vi "UpdateStatistics.vi"(8 "error in (no error)":errorcluster, 10 "Statistics":cluster{"OK":i32, "NG":i32}, 11 "WebSocket in":refnum<class "WebSocket.lvclass">) -> (0 "error out":errorcluster, 3 "WebSocket out":refnum<class "WebSocket.lvclass">)   [LabVIEW 2019, in "WebSocket.lvlib" / "WebSocket.lvclass"]
uses:
  WebSocket.lvclass
  ec31b149-a411-4443-9d0d-94b6aa8f2f4f.vi
  <vilib>/JDP Science/JSONtext/Variant to JSON Text.vi
  <vilib>/JDP Science/JSONtext/LVClass Serializer/JSONtext LVClass Serializer.lvclass
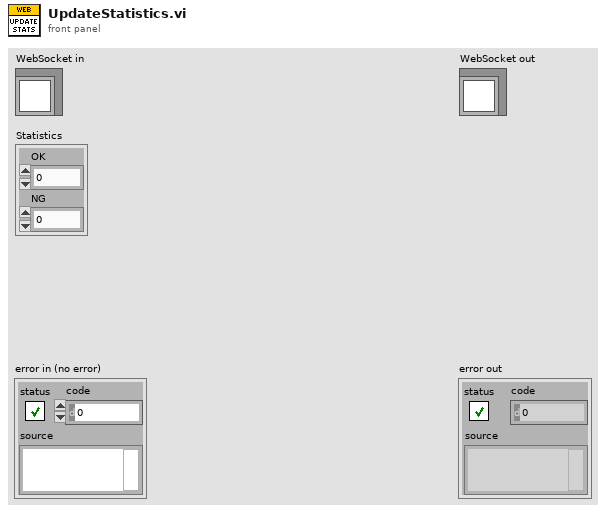
[diagram p1: front panel]
types:
  T1 = cluster{"type":string, "count":cluster{"ok":i32, "ng":i32, "yield":dbl}}
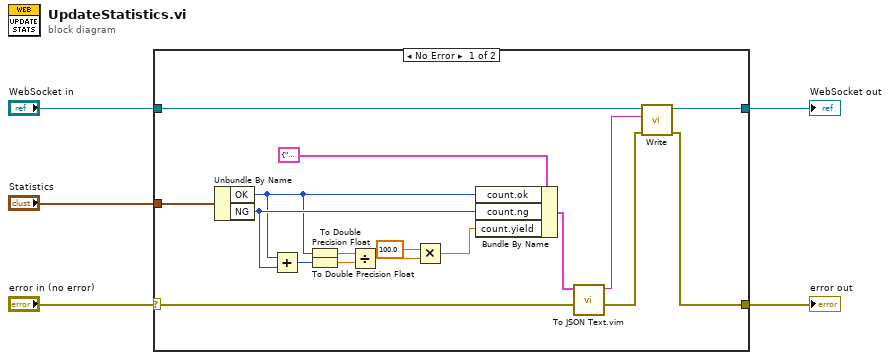
[diagram p0: block diagram]
diagram:
  n1 = case shown="No Error" "error in (no error)" {
    selector: "error in (no error)" -> [w17 w24]
    tunnel: [w14 w24] -> w4
    tunnel: [w21 w23] -> w2
    tunnel: "WebSocket in" -> [w22 w23]
    tunnel: "Statistics" -> [w19 _]
    frame No Error {
      n2 = Unbundle By Name(w19) -> ("OK"=w11:i32, "NG"=w13:i32)
      n3 = Add(x=w11, y=w13) -> (x+y=w12:i32)
      n4 = To Double Precision Float(number=w11) -> (double precision float=w9:dbl)
      n5 = To Double Precision Float(number=w12) -> (double precision float=w10:dbl)
      n6 = Divide(x=w9, y=w10) -> (x/y=w8:dbl)
      n7 = Multiply(x=100.0, y=w8) -> (x*y=w7:dbl)
      n8 = Bundle By Name(cluster=T1 {"type"="statistics", "count"={"ok"=0, "ng"=0, "yield"=0.0}}, "count.ok"=w11, "count.ng"=w13, "count.yield"=w7) -> (w18:T1)
      n9 = call "To JSON Text.vim"("error in (no error)"=w17, "Anything"=w18) -> ("error out"=w16:errorcluster, "<JSON>"=w15:string)  [unwired: 8 in]
      n10 = call "Write.vi"("error in (no error)"=w16, "Write"=w15, "WebSocket in"=w22) -> ("error out"=w14:errorcluster, "WebSocket out"=w21:refnum<class "WebSocket.lvclass">)  [unwired: 7 in]
    }
    frame Error {
    }
  }
  "error out" <- w4
  "WebSocket out" <- w2
